vi "Expand Special Cluster.vi"(6 "Special Term Indices In":T1={"Action"=-1, "Init"=-1, "Tag"=-1, "State in"=-1, "State out"=-1, "Error"=-1}, 9 "Starting TypeDesc":T2, 10 "Special Terminal":T5, 11 "Variant":variant) -> (0 "Save Types?":bool, 1 "Contained TypeDescs":T2[](array[typedef]), 4 "Special Term Indices":T1={"Action"=-1, "Init"=-1, "Tag"=-1, "State in"=-1, "State out"=-1, "Error"=-1})   [LabVIEW 2020, in "FlexBlocks.lvlib"]
uses:
  FlexBlocks.lvlib
  Special Terminal.ctl
  Type Descriptor.ctl
  Terminal Direction.ctl
  Value Mode.ctl
  Special Terminal Indices.ctl
  <vilib>/addons/analyzer/_analyzerutils.llb/VIAnUtil Check Type If ErrClust.vi
  <vilib>/Utility/Data Type/NI_Data Type.lvlib
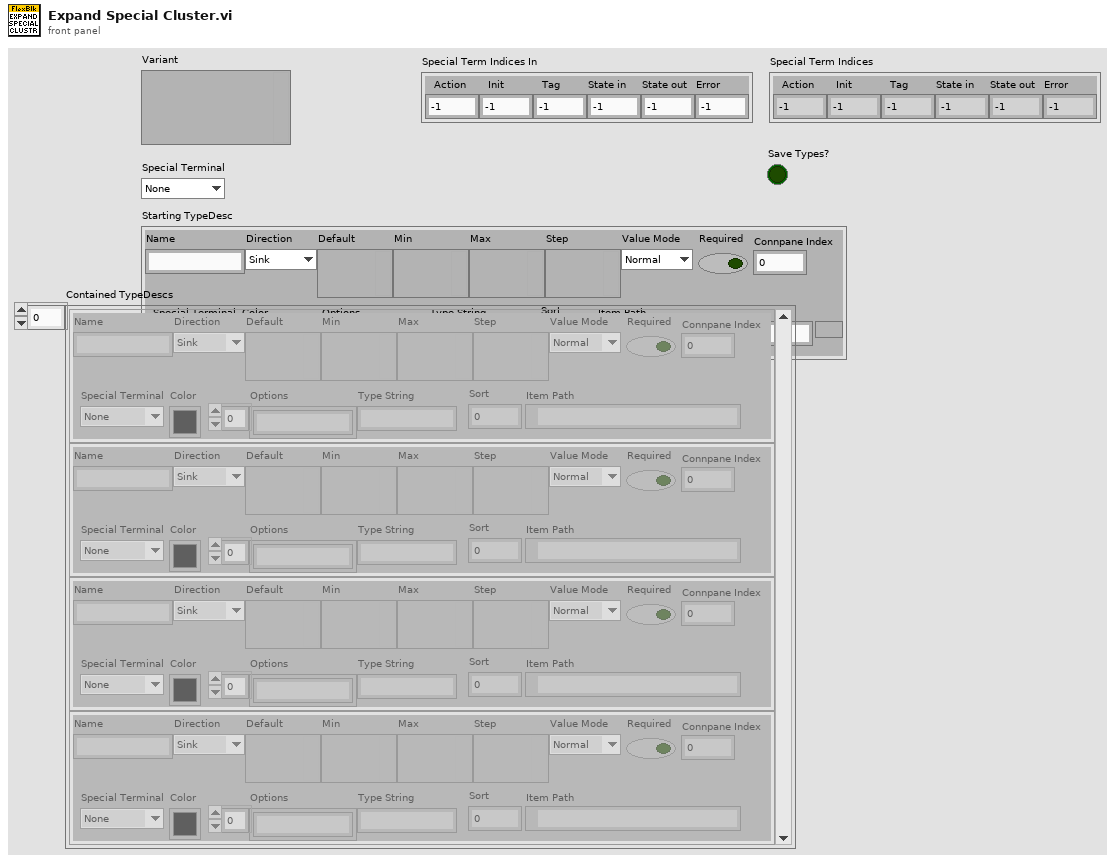
[diagram p1: front panel]
types:
  T1 = typedef "FlexBlocks.lvlib/Special Terminal Indices.ctl" = cluster{"Action":i32, "Init":i32, "Tag":i32, "State in":i32, "State out":i32, "Error":i32}
  T2 = typedef "FlexBlocks.lvlib/Type Descriptor.ctl" = cluster{"Name":string, "Direction":T3, "Default":variant, "Min":variant, "Max":variant, "Step":variant, "Value Mode":T4, "Required":bool, "Connpane Index":i32, "Special Terminal":T5, "Color":u32, "Options":string[], "Type String":string, "Sort":i32, "Item Path":path}
  T3 = typedef "FlexBlocks.lvlib/Terminal Direction.ctl" = enum16{"Sink", "Source"}
  T4 = typedef "FlexBlocks.lvlib/Value Mode.ctl" = enum16{"Normal", "Range", "Select"}
  T5 = typedef "FlexBlocks.lvlib/Special Terminal.ctl" = enum16{"None", "Action", "Init", "Tag", "State in", "State out", "Error"}
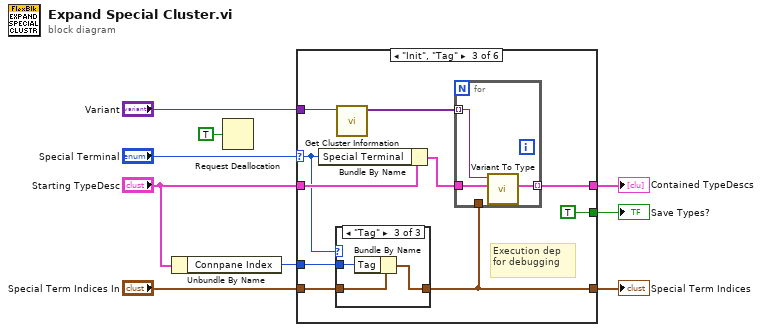
[diagram p0: block diagram]
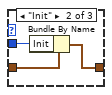
[diagram p5: hidden frame]
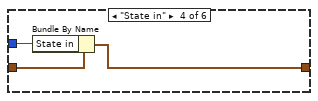
[diagram p6: hidden frame]
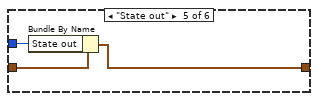
[diagram p7: hidden frame]
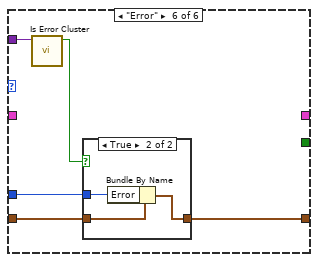
[diagram p8: hidden frame]
diagram:
  n1 = Unbundle By Name("Starting TypeDesc") -> ("Connpane Index"=w8:i32)
  n2 = Request Deallocation(TRUE ("flag")) -> ()
  n3 = case shown="\"Init\", \"Tag\"" "Special Terminal" {
    selector: "Special Terminal" -> [_ _ w16 _ _ _]
    tunnel: "Special Term Indices In" -> [w10 w11 w15 w34 w37 w41]
    tunnel: w8 -> [_ _ w17 w32 w35 w40]
    tunnel: "Starting TypeDesc" -> [_ _ w21 _ _ _]
    tunnel: [w10 w11 w12 w33 w36 w38] -> w5
    tunnel: "Variant" -> [_ _ w14 _ _ w42]
    tunnel: [_ _ w19 _ _ _] -> w2
    tunnel: [_ _ TRUE _ _ _] -> w1
    frame "None" {
    }
    frame "Action" {
    }
    frame "Init", "Tag" {
      # "Execution dep for debugging"
      n4 = Bundle By Name(cluster=w21, "Special Terminal"=w16) -> (w20:T2)
      n5 = case shown="\"Tag\"" w16 {
        tunnel: w17 -> [_ w24 w27]
        tunnel: w15 -> [w22 w25 w28]
        tunnel: [w22 w23 w26] -> w12
        frame Default {
        }
        frame "Init" {
          n6 = Bundle By Name(cluster=w25, "Init"=w24) -> (w23:T1)
        }
        frame "Tag" {
          n7 = Bundle By Name(cluster=w28, "Tag"=w27) -> (w26:T1)
        }
      }
      n8 = call <vilib>:"Get Cluster Information.vi"("variant"=w14) -> ("cluster elements"=w13:variant[])  [unwired: 9 in, 1 out]
      n9 = for {
        tunnel: w20 -> [w31]
        tunnel: [w30] -> w19 mode=indexing
        tunnel: w13 -> [w29] mode=indexing
        tunnel: w12 -> [_]
        n10 = call "Variant To Type.vi"("Type In"=w31, "Value"=w29) -> ("Type"=w30:T2)  [unwired: 9 in]
      }
    }
    frame "State in" {
      n11 = Bundle By Name(cluster=w34, "State in"=w32) -> (w33:T1)
    }
    frame "State out" {
      n12 = Bundle By Name(cluster=w37, "State out"=w35) -> (w36:T1)
    }
    frame "Error" {
      n13 = call <vilib>:"Is Error Cluster.vi"("variant"=w42) -> ("is error cluster?"=w39:bool)  [unwired: 9 in, 1 out]
      n14 = case shown="True" w39 {
        tunnel: w41 -> [w43 w46]
        tunnel: w40 -> [_ w45]
        tunnel: [w43 w44] -> w38
        frame False {
        }
        frame True {
          n15 = Bundle By Name(cluster=w46, "Error"=w45) -> (w44:T1)
        }
      }
    }
  }
  "Contained TypeDescs" <- w2
  "Special Term Indices" <- w5
  "Save Types?" <- w1
